vi "Generate_Data_Global.vi"() -> ()   [LabVIEW 2021]
doc: "Used to transfer the data from Generator_a to Aquisition_a."
panel:
  in  "Generate_Data_Global":dbl
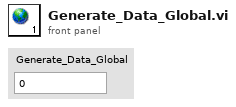
[diagram p1: front panel]
diagram:
